vi "Skyline Send Waveform File.vi"(8 "error in":errorcluster, 9 "properties":cluster{"Key":string, "Value":string}[](array[cluster]) caption="properties (null)", 11 "data in":waveform(dbl)[](array[waveform])) -> (0 "error out":errorcluster, 2 "size in bytes":i32)   [LabVIEW 2020, in "Logger.lvclass"]
uses:
  logger/Logger.lvclass
  <vilib>/Skyline/File/File/Send Buffer.vi
  <vilib>/Skyline/File/File/NI Skyline File.lvclass
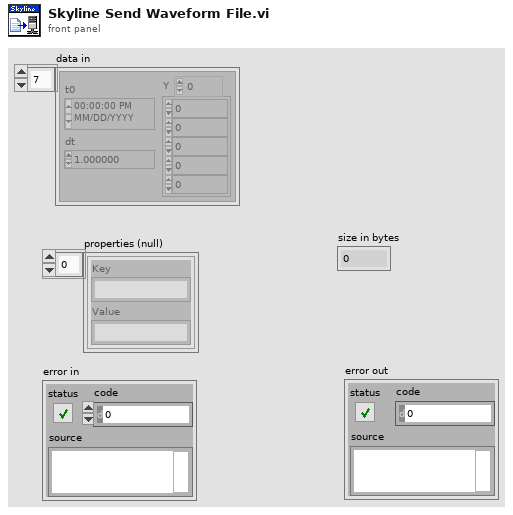
[diagram p1: front panel]
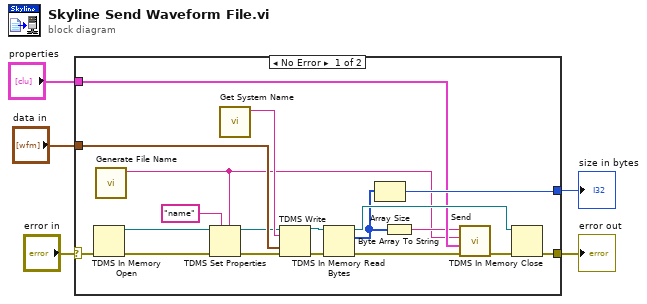
[diagram p0: block diagram]
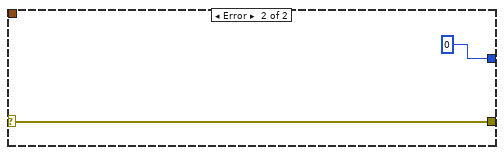
[diagram p2: hidden frame]
diagram:
  n1 = case shown="No Error" "error in" {
    selector: "error in" -> [w19 w26]
    tunnel: [w20 w26] -> w5
    tunnel: "properties" -> [w15 _]
    tunnel: "data in" -> [w24 _]
    tunnel: [w17 0] -> w1
    frame No Error {
      n2 = TDMS In Memory Open(8:w19) -> (0:w11:errorcluster, 3:w7:refnum<k34>)  [unwired: 1 in]
      n3 = call "Generate File Name.vi"() -> ("file name"=w9:string)  [unwired: 11 in]
      n4 = TDMS Set Properties(5:w9, 7:"name" ("property names"), 8:w11, 11:w7) -> (0:w10:errorcluster, 3:w6:refnum<k34>)  [unwired: 2 in, 2 out]
      n5 = call "Get System Name.vi"() -> ("name"=w16:string)  [unwired: 11 in]
      n6 = TDMS Write(0:w6, 5:w16, 9:w24, 11:w10) -> (4:w22:refnum<k34>, 15:w23:errorcluster)  [unwired: 2 in, 2 out]
      n7 = TDMS In Memory Read Bytes(8:w23, 11:w22) -> (0:w14:errorcluster, 2:w18:u8[], 3:w21:refnum<k34>)  [unwired: 2 in]
      n8 = Array Size(array=w18) -> (size(s)=w17:i32)
      n9 = Byte Array To String(unsigned byte array=w18) -> (string=w13:string)
      n10 = call-poly <vilib>:"Send.vi"("error in (no error)"=w14, "properties"=w15, "file name"=w9, "data"=w13) -> ("error out"=w12:errorcluster)  [unwired: 5 in, 1 out]
      n11 = TDMS In Memory Close(8:w12, 11:w21) -> (0:w20:errorcluster)  [unwired: 2 in]
    }
    frame Error {
    }
  }
  "error out" <- w5
  "size in bytes" <- w1
